vi "Disable FP Updates.vi"(8 "error in (no error)":errorcluster, 10 "Disable":bool, 11 "ViewableActor in":refnum<class "ViewableActor.lvclass">) -> (0 "error out":errorcluster, 3 "ViewableActor out":refnum<class "ViewableActor.lvclass">)   [LabVIEW 2020, in "ViewableActor.lvlib" / "ViewableActor.lvclass"]
uses:
  ViewableActor.lvclass
  ViewableActor.lvclass/ViewableActor.ctl
  Read UI VI Ref.vi
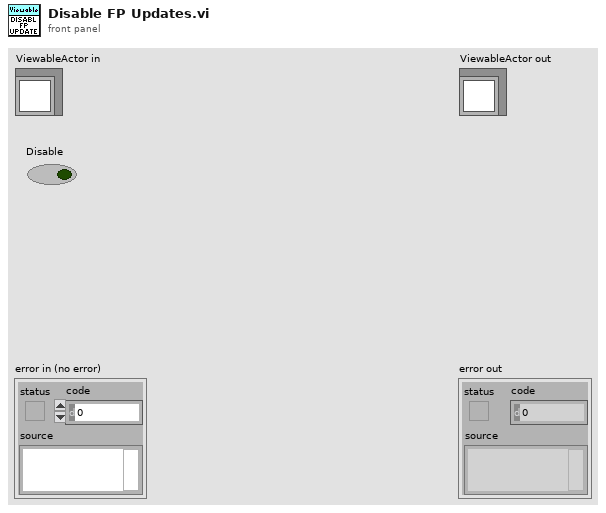
[diagram p1: front panel]
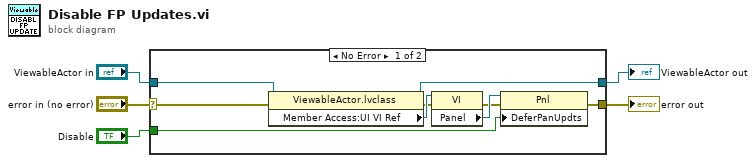
[diagram p0: block diagram]
diagram:
  n1 = case shown="No Error" "error in (no error)" {
    selector: "error in (no error)" -> [w7 w16]
    tunnel: [w6 w16] -> w2
    tunnel: [w13 w15] -> w1
    tunnel: "ViewableActor in" -> [w14 w15]
    tunnel: "Disable" -> [w10 _]
    frame No Error {
      n2 = property class="ViewableActor.lvclass"(reference=w14, error in=w7) -> (reference out=w13:refnum<class "ViewableActor.lvclass">, error out=w9:errorcluster, "Member Access:UI VI Ref"=w12:refnum<vi>)
      n3 = property class="VI"(reference=w12, error in=w9) -> (error out=w8:errorcluster, "Panel"=w11:refnum<vi>)  [unwired: 1 out]
      n4 = property class="Pnl"(reference=w11, error in=w8, "DeferPanUpdts"=w10) -> (error out=w6:errorcluster)  [unwired: 1 out]
    }
    frame Error {
    }
  }
  "error out" <- w2
  "ViewableActor out" <- w1
